vi "Application Data Directory.vi"(1 "Relative path (.)":path=path "") -> (0 "Application Directory (+ Relative)":path)   [LabVIEW 2013, in "Path Function.lvlib"]
doc: "Returns the LV App directory + Relative path."
uses:
  Path Function.lvlib
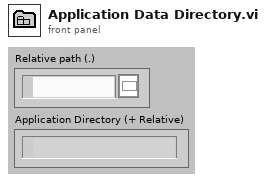
[diagram p1: front panel]
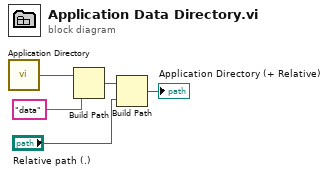
[diagram p0: block diagram]
diagram:
  n1 = call <vilib>:"Application Directory.vi"() -> ("Application Directory"=w1:path)
  n2 = Build Path(base path=w1, name or relative path="data" ("名称或相对路径")) -> (appended path=w3:path)
  n3 = Build Path(base path=w3, name or relative path="Relative path (.)") -> (appended path=→"Application Directory (+ Relative)":path)
